vi "Predict_Filenames_Generated.vi"(11 "Traverse line":T1 {"Carrier_2 Q (l/min)" format="%#.2f"; "Row Duration (mins)" format="%#.1f"; "Row No" min=0; "Trace Gas Concentration (%)" min=0.0 format="%#_4f"; "Carrier_1 Q (l/min)" format="%#.2f"; "Tunnel Speed" format="%#.2f"; "Start X" format="%#.2f"; "Start Y" format="%#.2f"; "Start Z" format="%#.2f"; "End X" format="%#.2f"; "End Y" format="%#.2f"; "End Z" format="%#.2f"; "Averaging time (min)" min=0.0 format="%#.2f"}) -> (3 "Filename":path[](array[path]))   [LabVIEW 2015]
uses:
  Gen Trav/Traverse_cluster.ctl
  Gen Trav/Spacing.ctl
  Controls/Multi_run_mode.ctl
panel:
  # "X           Y            Z"
  # "Start"
  # "End"
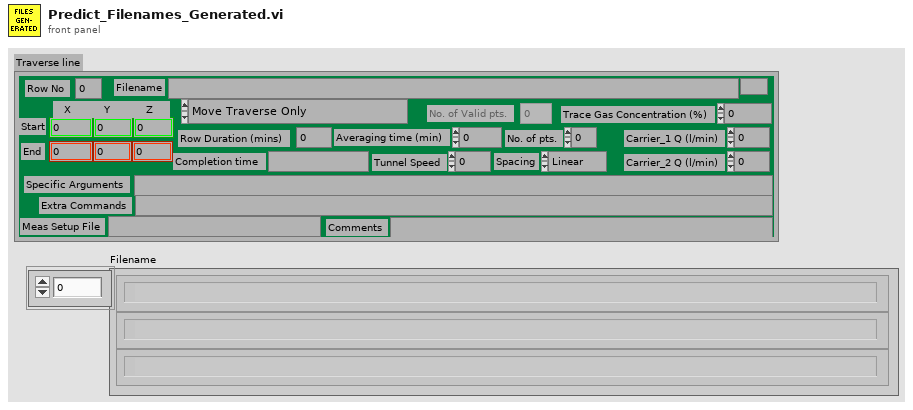
[diagram p1: front panel]
types:
  T1 = typedef "Traverse_cluster.ctl" = cluster{"Start X":sgl, "Start Y":sgl, "Start Z":sgl, "End X":sgl, "End Y":sgl, "End Z":sgl, "No. of pts.":i32, "Spacing":T2, "Filename":path, "Tunnel Speed":dbl, "Averaging time (min)":dbl, "Extra Commands":string, "Carrier_1 Q (l/min)":dbl, "Carrier_2 Q (l/min)":dbl, "Trace Gas Concentration (%)":dbl, "Specific Arguments":string, "Comments":string, "Row No":i32, "Row Type Selector":T3, "Completion time":string, "Row Duration (mins)":dbl, "No. of Valid pts.":i32, "Meas Setup File":string}
  T2 = typedef "Spacing.ctl" = enum16{"Linear", "Log", "Gauss", "Specified", "N/A"}
  T3 = typedef "Multi_run_mode.ctl" = enum16{"Move Traverse Only", "Set Tunnel Speed Only", "Set Source Only", "Set Measurement Conditions", "Single Measurement", "Vertical Profile", "Lateral Profile", "Longitudinal Profile", "Explore Volume", "Multi-Axis Profile", "Auto Calibrate", "Meas Fast FID Bkgnd", "Check Beam Power", "Scanning Valve Measurement", "Run VI Named:", "Set ADAM Ch", "Wait (minutes)", "Send Message", "Synchronize With:", "Fall Back to this Row", "Turn Off Row Repeating", "Blank Row", "Traverse 3D Volume"}
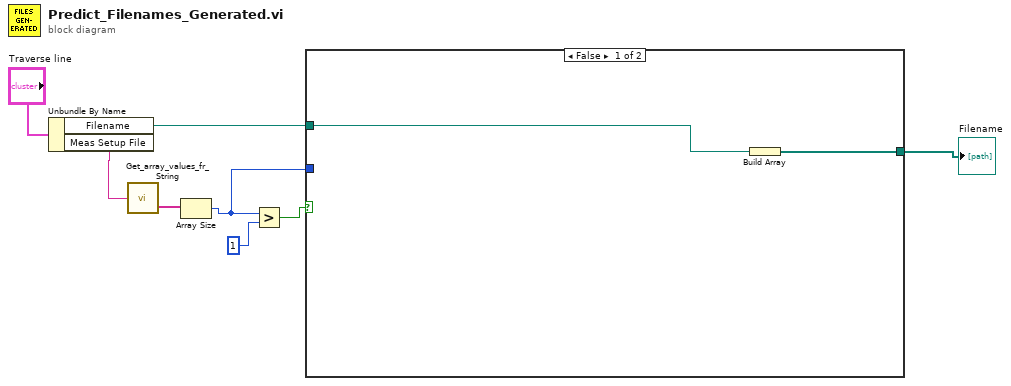
[diagram p0: block diagram]
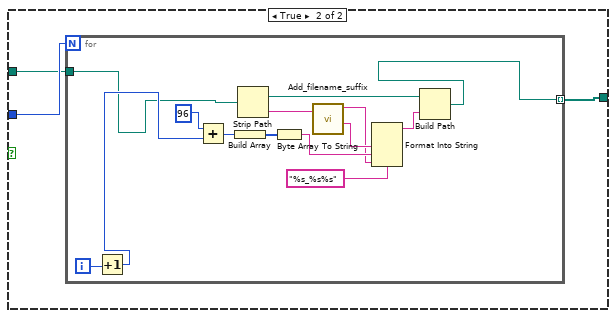
[diagram p2: hidden frame]
diagram:
  n1 = Unbundle By Name("Traverse line") -> ("Filename"=w2:path, "Meas Setup File"=w8:string)
  n2 = call "Get_array_values_fr_String.vi"("String Value"=w8) -> ("String array"=w6:string[])  [unwired: 1 out]
  n3 = Array Size(array=w6) -> (size(s)=w1:i32)
  n4 = Greater?(x=w1, y=1) -> (0:w4:bool)
  n5 = case shown="False" w4 {
    tunnel: [w9 w11] -> w3
    tunnel: w2 -> [w10 w12]
    tunnel: w1 -> [_ w13]
    frame False {
      n6 = Build Array(w10) -> (w9:path[])
    }
    frame True {
      n7 = for {
        N: w13 -> [_]
        tunnel: w12 -> [w25]
        tunnel: [w24] -> w11 mode=indexing
        i -> [w27]
        n8 = Increment(x=w27) -> (x+1=w26:i32)
        n9 = Add(x=96, y=w26) -> (x+y=w22:i32)
        n10 = Build Array(w22) -> (w23:i32[])
        n11 = Strip Path(path=w25) -> (stripped path=w15:path, name=w20:string)
        n12 = Byte Array To String(unsigned byte array=w23) -> (string=w18:string)
        n13 = call "Add_filename_suffix.vi"("Filename"=w20) -> ("Original Suffix"=w17:string, "Base name"=w19:string)  [unwired: 1 in, 2 out]
        n14 = Format Into String(format string="%s_%s%s", w19, w18, w17) -> (resulting string=w16:string)  [unwired: 2 in, 1 out]
        n15 = Build Path(base path=w15, name or relative path=w16) -> (appended path=w24:path)
      }
    }
  }
  "Filename" <- w3
